vi "clear.vi"(8 "error in (no error)":errorcluster, 11 "Measurement in":refnum<class "Measurement.lvclass">) -> (0 "error out":errorcluster, 3 "Measurement out":refnum<class "Measurement.lvclass">)   [LabVIEW 2017, in "Measurement.lvclass"]
doc: "Clear the measurement"
uses:
  Measurement.lvclass
  Measurement.lvclass/Measurement.ctl
  hardware/Hardware.lvclass
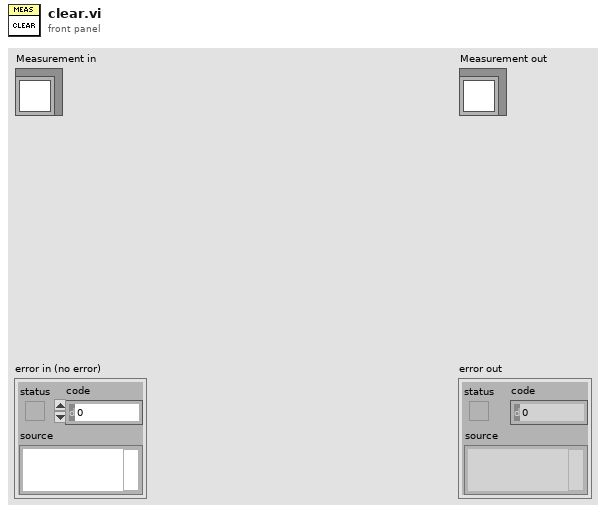
[diagram p1: front panel]
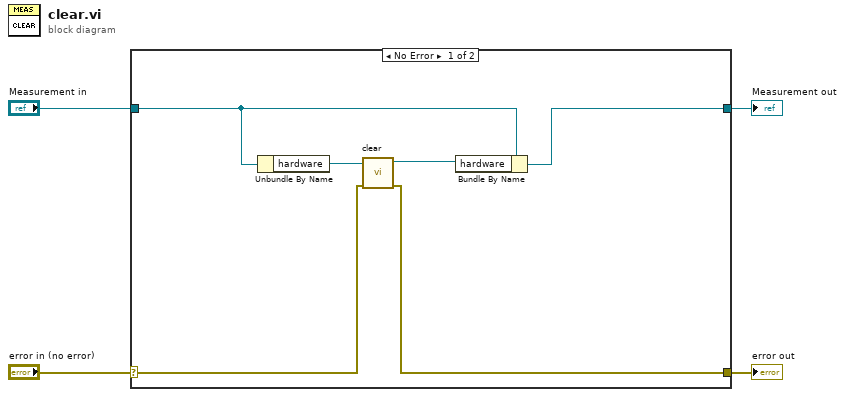
[diagram p0: block diagram]
diagram:
  n1 = case shown="No Error" "error in (no error)" {
    selector: "error in (no error)" -> [w6 w12]
    tunnel: [w5 w12] -> w3
    tunnel: [w8 w11] -> w1
    tunnel: "Measurement in" -> [w9 w11]
    frame No Error {
      n2 = Unbundle By Name(w9) -> ("hardware"=w10:refnum<class "Hardware.lvclass">)
      n3 = call-dynamic "clear.vi"("error in (no error)"=w6, "Hardware in"=w10) -> ("error out"=w5:errorcluster, "Hardware out"=w7:refnum<class "Hardware.lvclass">)  [unwired: 8 in]
      n4 = Bundle By Name(cluster=w9, "hardware"=w7) -> (w8:refnum<class "Measurement.lvclass">)
    }
    frame Error {
    }
  }
  "error out" <- w3
  "Measurement out" <- w1
